vi "Buzzer Music.vi"(0 "Boolean":bool) -> ()   [LabVIEW 2017]
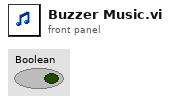
[diagram p1: front panel]
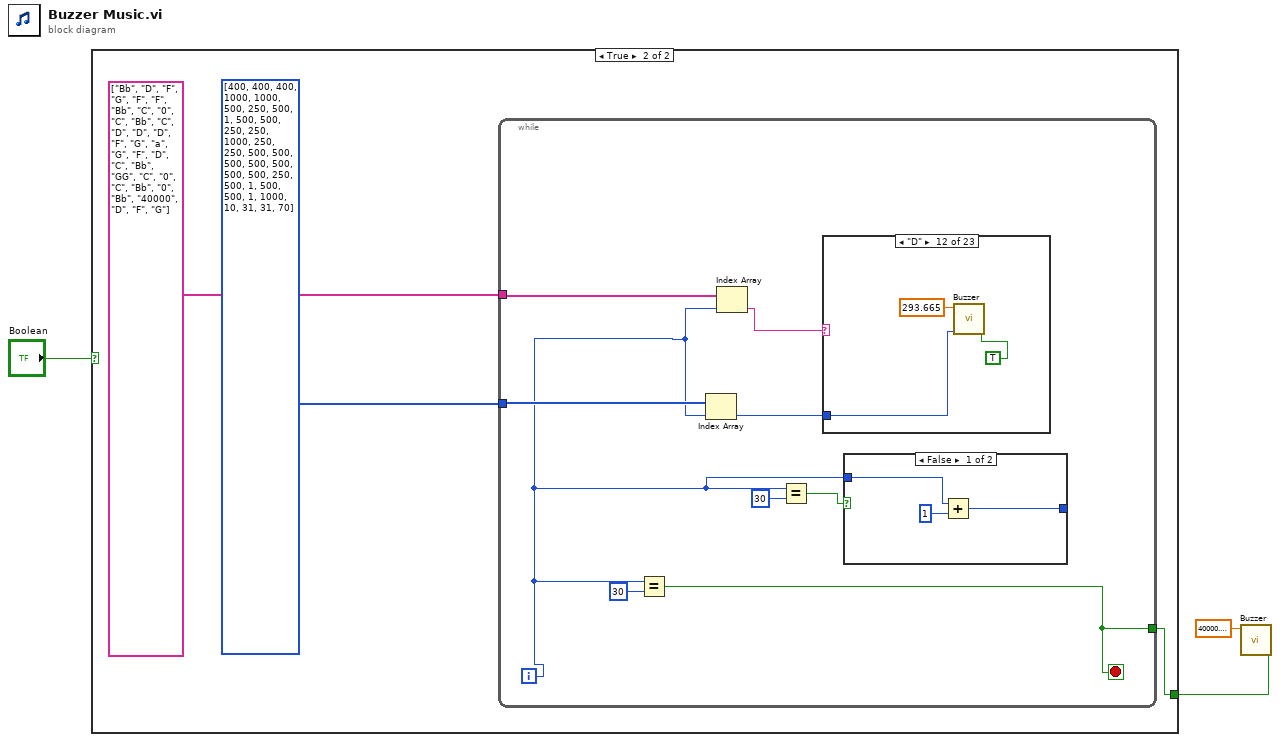
[diagram p0: block diagram]
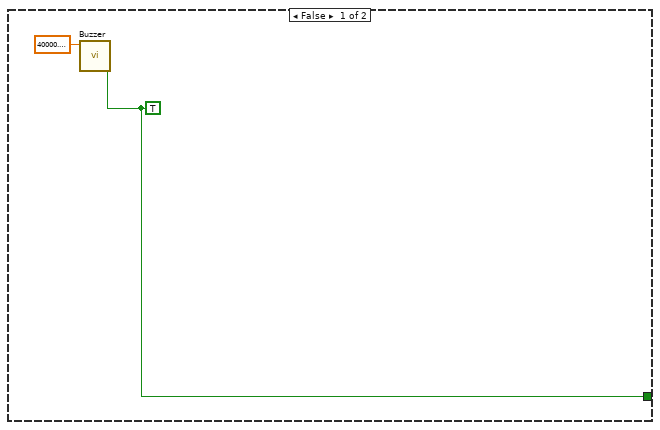
[diagram p2: hidden frame]
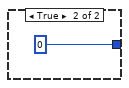
[diagram p3: hidden frame]
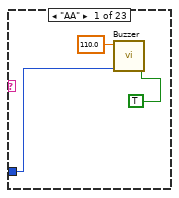
[diagram p4: hidden frame]
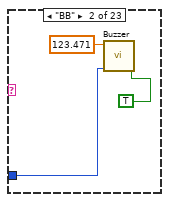
[diagram p5: hidden frame]
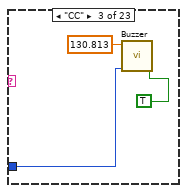
[diagram p6: hidden frame]
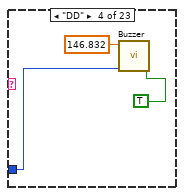
[diagram p7: hidden frame]
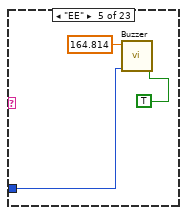
[diagram p8: hidden frame]
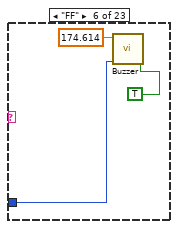
[diagram p9: hidden frame]
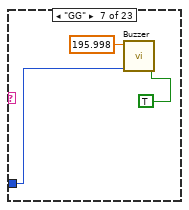
[diagram p10: hidden frame]
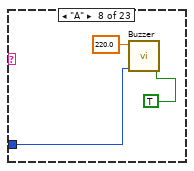
[diagram p11: hidden frame]
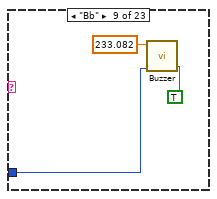
[diagram p12: hidden frame]
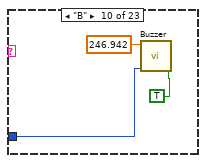
[diagram p13: hidden frame]
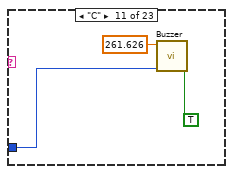
[diagram p14: hidden frame]
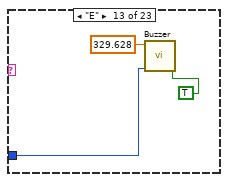
[diagram p15: hidden frame]
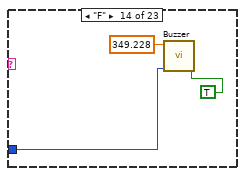
[diagram p16: hidden frame]
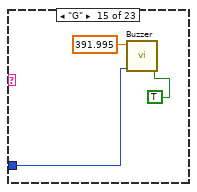
[diagram p17: hidden frame]
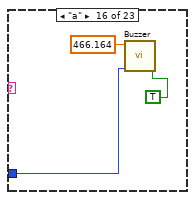
[diagram p18: hidden frame]
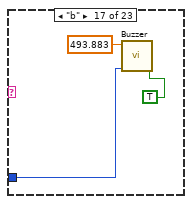
[diagram p19: hidden frame]
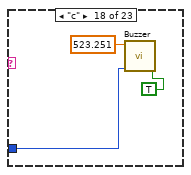
[diagram p20: hidden frame]
diagram:
  n1 = case shown="True" "Boolean" {
    tunnel: [w4 w6] -> w1
    frame False {
      w4 = TRUE ("[ESC]")
      n2 = call "Buzzer.vi"("[ESC]"=w4, "frequency [Hz]"=40000.000000000044) -> ()  [unwired: 10 in]
    }
    frame True {
      n3 = while {
        tunnel: i32[] [400, 400, 400, 1000, 1000, 500, 250, 500, 1, 500, 500, 250, 250, 1000, 250, 250, 500, 500, 500, 500, 500, 500, 500, 250, 500, 1, 500, 500, 1, 1000, 10, 31, 31, 70] -> [w17]
        tunnel: string[] ["Bb", "D", "F", "G", "F", "F", "Bb", "C", "0", "C", "Bb", "C", "D", "D", "D", "F", "G", "a", "G", "F", "D", "C", "Bb", "GG", "C", "0", "C", "Bb", "0", "Bb", "40000", "D", "F", "G"] -> [w14]
        tunnel: [w9] -> w6
        i -> [w11]
        stop <- w9 stop-if-true
        n4 = Equal?(x=w11, y=30) -> (x = y?=w9:bool)
        n5 = Index Array(array=w17, index=w11) -> (element=w16:i32)
        n6 = Index Array(array=w14, index=w11) -> (element=w12:string)
        n7 = Equal?(x=w11, y=30) -> (x = y?=w13:bool)
        n8 = case shown="\"D\"" w12 {
          tunnel: w16 -> [w22 w25 w28 w31 w34 w37 w40 w43 w46 w49 w52 w55 w58 w61 w64 w67 w70 w73 w76 w79 w82 w85 w89]
          frame "AA" {
            n9 = call "Buzzer.vi"("[ESC]"=TRUE, "milliseconds to wait"=w22, "frequency [Hz]"=110.0) -> ()  [unwired: 9 in]
          }
          frame "BB" {
            n10 = call "Buzzer.vi"("[ESC]"=TRUE, "milliseconds to wait"=w25, "frequency [Hz]"=123.471) -> ()  [unwired: 9 in]
          }
          frame "CC" {
            n11 = call "Buzzer.vi"("[ESC]"=TRUE, "milliseconds to wait"=w28, "frequency [Hz]"=130.813) -> ()  [unwired: 9 in]
          }
          frame "DD" {
            n12 = call "Buzzer.vi"("[ESC]"=TRUE, "milliseconds to wait"=w31, "frequency [Hz]"=146.832) -> ()  [unwired: 9 in]
          }
          frame "EE" {
            n13 = call "Buzzer.vi"("[ESC]"=TRUE, "milliseconds to wait"=w34, "frequency [Hz]"=164.814) -> ()  [unwired: 9 in]
          }
          frame "FF" {
            n14 = call "Buzzer.vi"("[ESC]"=TRUE, "milliseconds to wait"=w37, "frequency [Hz]"=174.614) -> ()  [unwired: 9 in]
          }
          frame "GG" {
            n15 = call "Buzzer.vi"("[ESC]"=TRUE, "milliseconds to wait"=w40, "frequency [Hz]"=195.998) -> ()  [unwired: 9 in]
          }
          frame "A" {
            n16 = call "Buzzer.vi"("[ESC]"=TRUE, "milliseconds to wait"=w43, "frequency [Hz]"=220.0) -> ()  [unwired: 9 in]
          }
          frame "Bb" {
            n17 = call "Buzzer.vi"("[ESC]"=TRUE, "milliseconds to wait"=w46, "frequency [Hz]"=233.082) -> ()  [unwired: 9 in]
          }
          frame "B" {
            n18 = call "Buzzer.vi"("[ESC]"=TRUE, "milliseconds to wait"=w49, "frequency [Hz]"=246.942) -> ()  [unwired: 9 in]
          }
          frame "C" {
            n19 = call "Buzzer.vi"("[ESC]"=TRUE, "milliseconds to wait"=w52, "frequency [Hz]"=261.626) -> ()  [unwired: 9 in]
          }
          frame "D" {
            n20 = call "Buzzer.vi"("[ESC]"=TRUE, "milliseconds to wait"=w55, "frequency [Hz]"=293.665) -> ()  [unwired: 9 in]
          }
          frame "E" {
            n21 = call "Buzzer.vi"("[ESC]"=TRUE, "milliseconds to wait"=w58, "frequency [Hz]"=329.628) -> ()  [unwired: 9 in]
          }
          frame "F" {
            n22 = call "Buzzer.vi"("[ESC]"=TRUE, "milliseconds to wait"=w61, "frequency [Hz]"=349.228) -> ()  [unwired: 9 in]
          }
          frame "G" {
            n23 = call "Buzzer.vi"("[ESC]"=TRUE, "milliseconds to wait"=w64, "frequency [Hz]"=391.995) -> ()  [unwired: 9 in]
          }
          frame "a" {
            n24 = call "Buzzer.vi"("[ESC]"=TRUE, "milliseconds to wait"=w67, "frequency [Hz]"=466.164) -> ()  [unwired: 9 in]
          }
          frame "b" {
            n25 = call "Buzzer.vi"("[ESC]"=TRUE, "milliseconds to wait"=w70, "frequency [Hz]"=493.883) -> ()  [unwired: 9 in]
          }
          frame "c" {
            n26 = call "Buzzer.vi"("[ESC]"=TRUE, "milliseconds to wait"=w73, "frequency [Hz]"=523.251) -> ()  [unwired: 9 in]
          }
          frame "d" {
            n27 = call "Buzzer.vi"("[ESC]"=TRUE, "milliseconds to wait"=w76, "frequency [Hz]"=587.33) -> ()  [unwired: 9 in]
          }
          frame "e" {
            n28 = call "Buzzer.vi"("[ESC]"=TRUE, "milliseconds to wait"=w79, "frequency [Hz]"=659.225) -> ()  [unwired: 9 in]
          }
          frame "f" {
            n29 = call "Buzzer.vi"("[ESC]"=TRUE, "milliseconds to wait"=w82, "frequency [Hz]"=698.456) -> ()  [unwired: 9 in]
          }
          frame "g" {
            n30 = call "Buzzer.vi"("[ESC]"=TRUE, "milliseconds to wait"=w85, "frequency [Hz]"=783.991) -> ()  [unwired: 9 in]
          }
          frame "0", Default {
            n31 = call "Buzzer.vi"("[ESC]"=TRUE, "milliseconds to wait"=w89, "frequency [Hz]"=0.0) -> ()  [unwired: 9 in]
          }
        }
        n32 = case shown="False" w13 {
          tunnel: w11 -> [w20 _]
          tunnel: [w18 0] -> _
          frame False {
            n33 = Add(x=w20, y=1) -> (x+y=w18:i32)
          }
          frame True {
          }
        }
      }
    }
  }
  n34 = call "Buzzer.vi"("[ESC]"=w1, "frequency [Hz]"=40000.000000000044) -> ()  [unwired: 10 in]
